vi "Add Item to Group.vi"(8 "error in (no error)":errorcluster, 10 "Menu Path":string, 11 "Selector in":refnum<class "Selector.lvclass">) -> (0 "error out":errorcluster, 1 "Group":string, 2 "Name":string, 3 "Selector out":refnum<class "Selector.lvclass">)   [LabVIEW 2019, in "Selector.lvclass"]
uses:
  Selector.lvclass
  Selector.lvclass/Selector.ctl
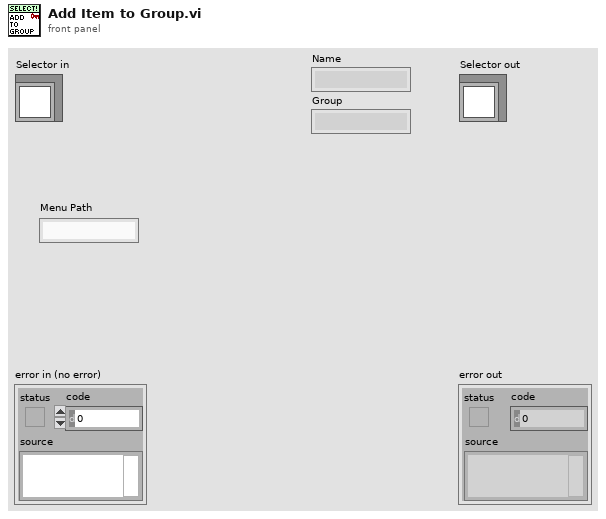
[diagram p1: front panel]
types:
  T1 = typedef "Selector.lvclass/Item.ctl" = cluster{"Name":string, "Group":string, "Enabled":bool}
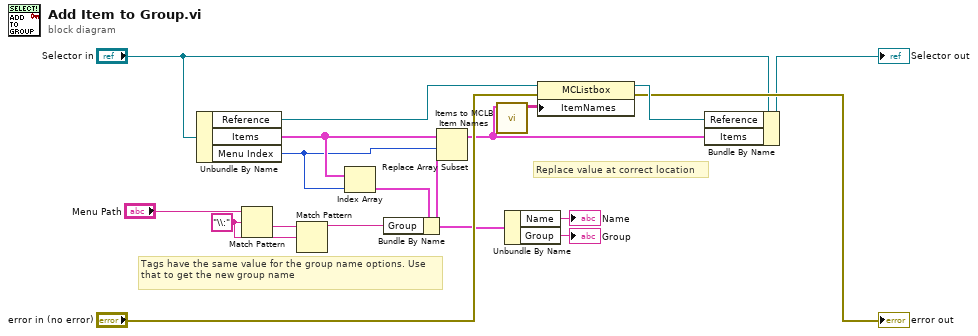
[diagram p0: block diagram]
diagram:
  w10 = "\\:" ("regular expression")
  # "Replace value at correct location"
  # "Tags have the same value for the group name options. Use that to get the new group name"
  n1 = Unbundle By Name("Selector in") -> ("Reference"=w16:refnum<vi>, "Items"=w8:T1[], "Menu Index"=w7:i32)
  n2 = Match Pattern(string="Menu Path", regular expression=w10) -> (after substring=w11:string)  [unwired: 1 in, 3 out]
  n3 = Match Pattern(string=w11, regular expression=w10) -> (before substring=w5:string)  [unwired: 1 in, 3 out]
  n4 = Index Array(array=w8, index=w7) -> (element=w6:T1)
  n5 = Bundle By Name(cluster=w6, "Group"=w5) -> (w3:T1)
  n6 = Replace Array Subset(array=w8, new element=w3, index=w7) -> (w4:T1[])
  n7 = call "Items to MCLB Item Names.vi"("Items"=w4) -> ("Item Names"=w9:string[][])  [unwired: 6 in]
  n8 = Unbundle By Name(w3) -> ("Name"=→"Name":string, "Group"=→"Group":string)
  n9 = property class="MCListbox"(reference=w16, error in="error in (no error)", "ItemNames"=w9) -> (reference out=w17:refnum<vi>, error out=→"error out":errorcluster)
  n10 = Bundle By Name(cluster="Selector in", "Reference"=w17, "Items"=w4) -> (→"Selector out":refnum<class "Selector.lvclass">)
